vi "error_filter.vi"(7 "Error Enum in":T1=enum."VISA_err_Timeout", 8 "error in":errorcluster caption="error in (no error)", 10 "Clear detected code (F)":bool, 11 "VISA resource name":refnum<visa-resource-name>) -> (0 "error out":errorcluster, 2 "Code Detected":bool, 3 "VISA resource name out":refnum<visa-resource-name>)   [LabVIEW 2022 SP3, in "hmp4000_rsidr_core.lvlib"]
uses:
  hmp4000_rsidr_core.lvlib
  type_Error_Codes.ctl
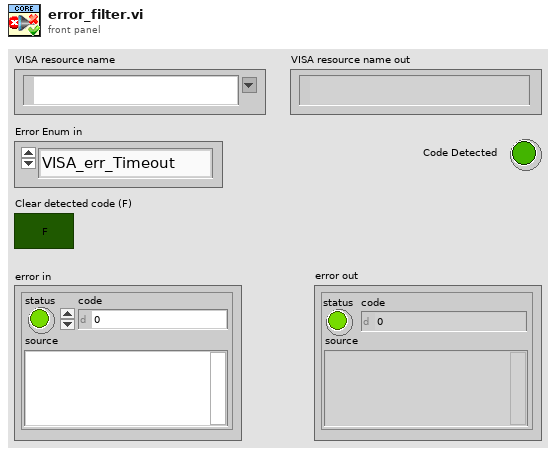
[diagram p1: front panel]
types:
  T1 = typedef "hmp4000_rsidr_core.lvlib/type_Error_Codes.ctl" = enum16{"No_error", "VISA_err_ResourceNotFound", "VISA_err_Timeout", "VISA_warn_MoreDataAvailable", "RS_err_MissingCallback", "RS_err_InvalidAttribute", "RS_err_InvalidValue", "RS_err_UnknownResource", "RS_err_AlreadyInitialized", "RS_err_InstrumentStatus", "RS_err_BadRepCapName", "RS_err_TypesMismatch", "RS_err_ValueNotSupported", "RS_err_InvalidRngTable", "RS_err_IDqueryFail", "RS_err_UnexpResponse", "VISA_warn_ConfigNotLoaded", "RS_err_AttributeNotReadable", "RS_err_AttributeNotWritable", "RS_err_InstrumentType", "RS_err_InstrumentOption", "VISA_err_InvalidSize", "RS_err_ReliabilityIndicator", "VISA_warn_UnknownStatus", "VISA_warn_TermCharRead", "VISA_err_IO_error", "RS_err_FunctionNotSupported", "VISA_warn_QueueEmpty"}
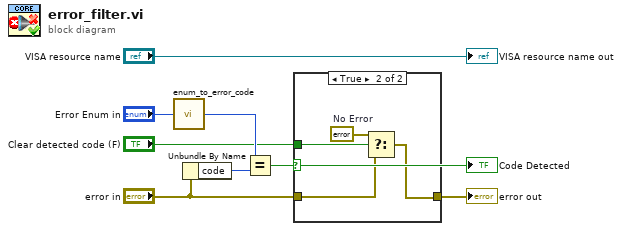
[diagram p0: block diagram]
diagram:
  n1 = call "enum_to_error_code.vi"("Error Enum in"="Error Enum in") -> ("error code out"=w3:i32)  [unwired: 4 in]
  n2 = Unbundle By Name("error in") -> ("code"=w8:i32)
  n3 = Equal?(x=w3, y=w8) -> (x = y?=w6:bool)
  "Code Detected" <- w6
  n4 = case shown="True" w6 {
    tunnel: "error in" -> [w9 w11]
    tunnel: [w9 w13] -> w5
    tunnel: "Clear detected code (F)" -> [_ w10]
    frame False {
    }
    frame True {
      w12 = errorcluster {"status"=FALSE, "code"=0, "source"=""}  # No Error
      n5 = Select(t=w12, s=w10, f=w11) -> (s? t:f=w13:errorcluster)
    }
  }
  "error out" <- w5
  "VISA resource name out" <- "VISA resource name"
